vi "KeithleyInit.vi"(8 "error in (no error)":errorcluster, 10 "SourceFunction":enum32{"Current", "Voltage"}(ring)=enum."Voltage", 11 "VISA Refnum in":refnum<visa-resource-name>) -> (0 "error out":errorcluster, 2 "Node Out":string, 3 "VISA Refnum out":refnum<visa-resource-name>)   [LabVIEW 2017]
uses:
  Keithley 2600 Series/Public/Channel.ctl
  Keithley 2600 Series/Keithley 2600 Series.lvlib
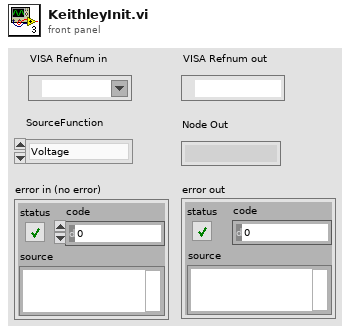
[diagram p1: front panel]
types:
  T1 = typedef "Keithley 2600 Series.lvlib/Channel.ctl" = enum32{"Channel A", "Channel B"}
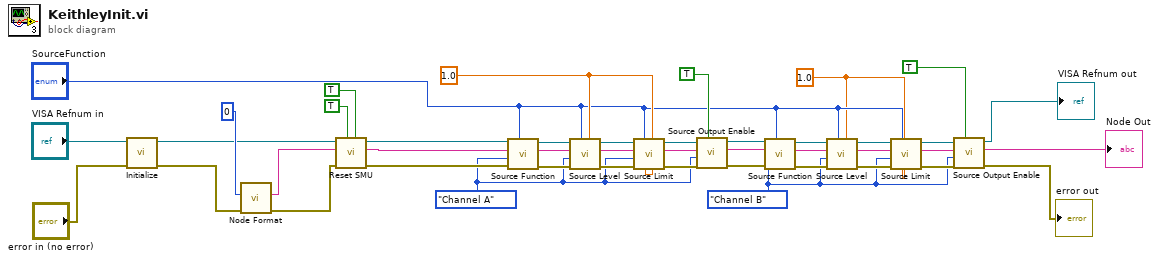
[diagram p0: block diagram]
diagram:
  w5 = 1.0 ("Level (0.000)")
  w6 = Channel."Channel B" ("Channel (Channel A)")
  w12 = Channel."Channel A" ("Channel (Channel A)")
  w36 = 1.0 ("Level (0.000)")
  n1 = call "Initialize.vi"("error in (no error)"="error in (no error)", "VISA resource name"="VISA Refnum in") -> ("error out"=w24:errorcluster, "VISA resource name out"=w25:refnum<visa-resource-name>)  [unwired: 8 in]
  n2 = call "Node Format.vi"("error in"=w24, "Node (0-64)"=i8 0) -> ("error out"=w27:errorcluster, "Formatted Node"=w26:string)  [unwired: 8 in]
  n3 = call "Reset SMU.vi"("SMU B (No)"=TRUE, "SMU A (No)"=TRUE, "error in (no error)"=w27, "Node In"=w26, "VISA resource name"=w25) -> ("error out"=w42:errorcluster, "Node Out"=w43:string, "VISA resource name out"=w41:refnum<visa-resource-name>)  [unwired: 4 out]
  n4 = call "Source Function.vi"("Function (Current)"="SourceFunction", "error in (no error)"=w42, "Channel (Channel A)"=w12, "Node In"=w43, "VISA resource name"=w41) -> ("error out"=w32:errorcluster, "Node Out"=w30:string, "VISA resource name out"=w31:refnum<visa-resource-name>)  [unwired: 4 out]
  n5 = call "Source Level.vi"("Level (0.000)"=w36, "Function (Current)"="SourceFunction", "error in (no error)"=w32, "Channel (Channel A)"=w12, "Node In"=w30, "VISA resource name"=w31) -> ("error out"=w33:errorcluster, "Node Out"=w35:string, "VISA resource name out"=w34:refnum<visa-resource-name>)  [unwired: 3 out]
  n6 = call "Source Limit.vi"("Limit (0.000)"=w36, "Function (Current)"="SourceFunction", "error in (no error)"=w33, "Channel (Channel A)"=w12, "Node In"=w35, "VISA resource name"=w34) -> ("error out"=w39:errorcluster, "Node Out"=w38:string, "VISA resource name out"=w37:refnum<visa-resource-name>)  [unwired: 3 out]
  n7 = call "Source Output Enable.vi"("Output (Off)"=TRUE, "error in (no error)"=w39, "Channel (Channel A)"=w12, "Node In"=w38, "VISA resource name"=w37) -> ("error out"=w10:errorcluster, "Node Out"=w9:string, "VISA resource name out"=w11:refnum<visa-resource-name>)  [unwired: 4 out]
  n8 = call "Source Function.vi"("Function (Current)"="SourceFunction", "error in (no error)"=w10, "Channel (Channel A)"=w6, "Node In"=w9, "VISA resource name"=w11) -> ("error out"=w15:errorcluster, "Node Out"=w13:string, "VISA resource name out"=w14:refnum<visa-resource-name>)  [unwired: 4 out]
  n9 = call "Source Level.vi"("Level (0.000)"=w5, "Function (Current)"="SourceFunction", "error in (no error)"=w15, "Channel (Channel A)"=w6, "Node In"=w13, "VISA resource name"=w14) -> ("error out"=w16:errorcluster, "Node Out"=w18:string, "VISA resource name out"=w17:refnum<visa-resource-name>)  [unwired: 3 out]
  n10 = call "Source Limit.vi"("Limit (0.000)"=w5, "Function (Current)"="SourceFunction", "error in (no error)"=w16, "Channel (Channel A)"=w6, "Node In"=w18, "VISA resource name"=w17) -> ("error out"=w21:errorcluster, "Node Out"=w20:string, "VISA resource name out"=w19:refnum<visa-resource-name>)  [unwired: 3 out]
  n11 = call "Source Output Enable.vi"("Output (Off)"=TRUE, "error in (no error)"=w21, "Channel (Channel A)"=w6, "Node In"=w20, "VISA resource name"=w19) -> ("error out"=→"error out":errorcluster, "Node Out"=→"Node Out":string, "VISA resource name out"=→"VISA Refnum out":refnum<visa-resource-name>)  [unwired: 4 out]
